vi "DateTimeString_to_TimeStamp.vi"(8 "error in":errorcluster, 11 "%m/%d/%Y %H:%M:%S string":string) -> (0 "error out":errorcluster, 3 "Time Stamp":timestamp)   [LabVIEW 2012]
doc: "This VI convert a date/time string back to a time stamp."
panel:
  # "This control should have data in the form:\n4/30/2004 7:48:47"
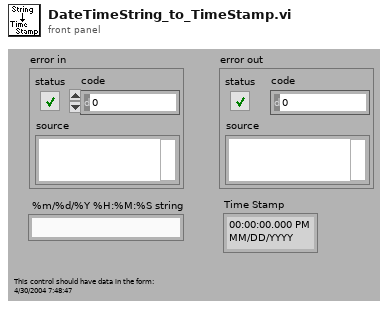
[diagram p1: front panel]
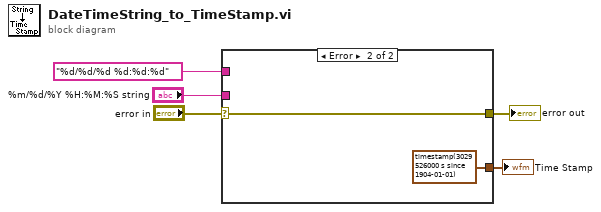
[diagram p0: block diagram]
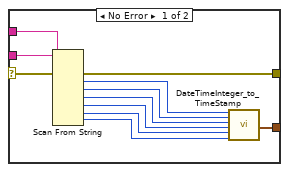
[diagram p2: hidden frame]
diagram:
  n1 = case shown="Error" "error in" {
    selector: "error in" -> [w6 w17]
    tunnel: "%m/%d/%Y %H:%M:%S string" -> [w16 _]
    tunnel: "%d/%d/%d %d:%d:%d" ("format string") -> [w15 _]
    tunnel: [w14 w17] -> w3
    tunnel: [w13 timestamp(3029526000 s since 1904-01-01) ("Time Stamp")] -> w2
    frame No Error {
      n2 = Scan From String(format string=w15, input string=w16, error in=w6) -> (error out=w14:errorcluster, output 1=w12:i32, output 2=w11:i32, output 3=w10:i32, output 4=w9:i32, output 5=w8:i32, output 6=w7:i32)  [unwired: 7 in, 2 out]
      n3 = call "DateTimeInteger_to_TimeStamp.vi"("Month"=w12, "Day of Month"=w11, "Year"=w10, "Hour"=w9, "Minute"=w8, "Second"=w7) -> ("Time Stamp"=w13:timestamp)  [unwired: 13 in]
    }
    frame Error {
    }
  }
  "Time Stamp" <- w2
  "error out" <- w3
